vi "Configure Checkweighing Threshold.vi"(8 "error in (no error)":errorcluster, 9 "Lower Limit(T)/Upper Limit (F)":bool, 10 "Threshold Value [g]":dbl, 11 "VISA resource name":refnum<visa-resource-name>) -> (0 "error out":errorcluster, 3 "VISA resource name out":refnum<visa-resource-name>)   [LabVIEW 2017, in "RadWag balances and scales.lvlib"]
doc: "This VI is used to set the thresholds values in chceckweighting mode.\nThis VI works properly when balance works in chceckweighting mode. (To configure work mode use Utility -> Set operating mode)"
uses:
  <instrlib>/Radwag Balances and Scales/Public/RadWag balances and scales.lvlib
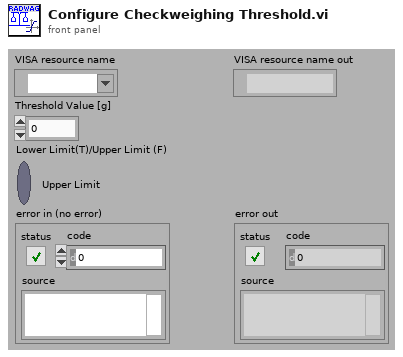
[diagram p1: front panel]
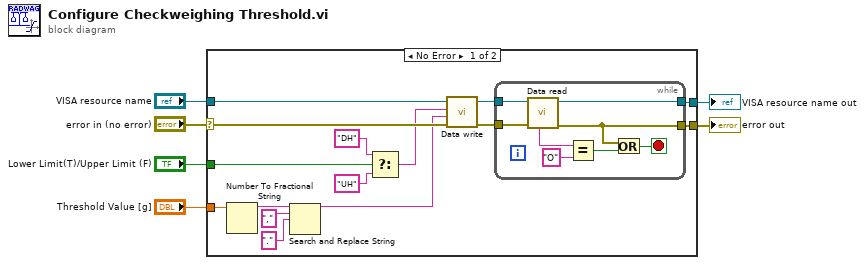
[diagram p0: block diagram]
diagram:
  n1 = case shown="No Error" "error in (no error)" {
    selector: "error in (no error)" -> [w12 w30]
    tunnel: "Threshold Value [g]" -> [w16 _]
    tunnel: "Lower Limit(T)/Upper Limit (F)" -> [w10 _]
    tunnel: "VISA resource name" -> [w15 w31]
    tunnel: [w14 w31] -> w2
    tunnel: [w13 w30] -> w1
    frame No Error {
      n2 = Number To Fractional String(number=w16) -> (F-format string=w17:string)  [unwired: 3 in]
      n3 = Search and Replace String(input string=w17, search string=",", replace string="." ("replace string (\"\")")) -> (result string=w11:string)  [unwired: 5 in, 3 out]
      n4 = Select(t="DH" ("ID"), s=w10, f="UH" ("ID")) -> (s? t:f=w7:string)
      n5 = call <instrlib>:"Data write.vi"("error in (no error)"=w12, "Parameter"=w11, "ID"=w7, "VISA resource name"=w15) -> ("error out"=w20:errorcluster, "VISA resource name out"=w21:refnum<visa-resource-name>)  [unwired: 6 in]
      n6 = while {
        tunnel: w21 -> [w29]
        tunnel: w20 -> [w28]
        tunnel: [w27] -> w14
        tunnel: [w22] -> w13
        stop <- w23 stop-if-true
        n7 = call <instrlib>:"Data read.vi"("error in (no error)"=w28, "VISA resource name"=w29) -> ("error out"=w22:errorcluster, "VISA resource name out"=w27:refnum<visa-resource-name>, "Status"=w26:string)  [unwired: 3 in, 4 out]
        n8 = Equal?(x=w26, y="O") -> (x = y?=w24:bool)
        n9 = Or(x=w22, y=w24) -> (x .or. y?=w23:bool)
      }
    }
    frame Error {
    }
  }
  "VISA resource name out" <- w2
  "error out" <- w1
